vi "DK240 Write.vi"(2 "error in":errorcluster, 3 "String to write":string, 4 "Port":refnum<visa-resource-name>="SPECTRO") -> (0 "error out":errorcluster)   [LabVIEW 2019]
doc: "Ce VI écrit la chaîne de commande indiquée sur le port série spécifié."
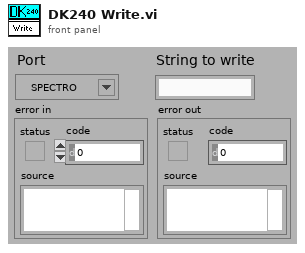
[diagram p1: front panel]
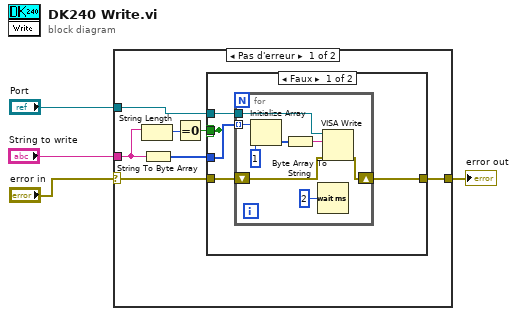
[diagram p0: block diagram]
diagram:
  n1 = case shown="Pas d'erreur" "error in" {
    selector: "error in" -> [w5 w25]
    tunnel: "String to write" -> [w8 _]
    tunnel: "Port" -> [w7 _]
    tunnel: [w6 w25] -> w3
    frame No Error {
      n2 = String Length(string=w8) -> (length=w11:i32)
      n3 = String To Byte Array(string=w8) -> (unsigned byte array=w9:u8[])
      n4 = Equal To 0?(x=w11) -> (x = 0?=w10:bool)
      n5 = case shown="Faux" w10 {
        tunnel: w10 -> [_ _]
        tunnel: w9 -> [w15 _]
        tunnel: w7 -> [w14 _]
        tunnel: w5 -> [w13 w24]
        tunnel: [w12 w24] -> w6
        frame False {
          n6 = for {
            tunnel: w15 -> [w21] mode=indexing
            tunnel: w14 -> [w18]
            shift-right: [w17] -> w12
            shift-left: w13 -> [w16]
            n7 = Initialize Array(w21, 1) -> (w20:u8[])
            n8 = Byte Array To String(unsigned byte array=w20) -> (string=w19:string)
            n9 = Wait (ms)(milliseconds to wait=2) -> ()  [unwired: 1 out]
            n10 = VISA Write(VISA resource name=w18, write buffer=w19, error in (no error)=w16) -> (error out=w17:errorcluster)  [unwired: 2 out]
          }
        }
        frame True {
        }
      }
    }
    frame Error {
    }
  }
  "error out" <- w3
